vi "Correggi database tempo acq da hms.vi"() -> ()   [LabVIEW 2019]
uses:
  <vilib>/addons/database/Connection.llb/Conn Execute.vi
  <vilib>/addons/database/Recordset.llb/Rec Fetch Recordset Data (R).vi
  <vilib>/addons/database/Recordset.llb/Rec Destroy - Connection.vi
  <vilib>/addons/database/_DB Variant To Data/Database Variant To Data.xnode
  <vilib>/addons/database/NI_Database_API.lvlib
panel:
  in  "Tempo T\\corrente F":bool
  out "data 2":string[][](array[string])
  out "Numeric 2":i32
  out "concatenated string 2":string
  out "error out 2":errorcluster
  out "error out":errorcluster
  out "concatenated string":string
  out "Numeric":i32
  out "data":string[][](array[string])
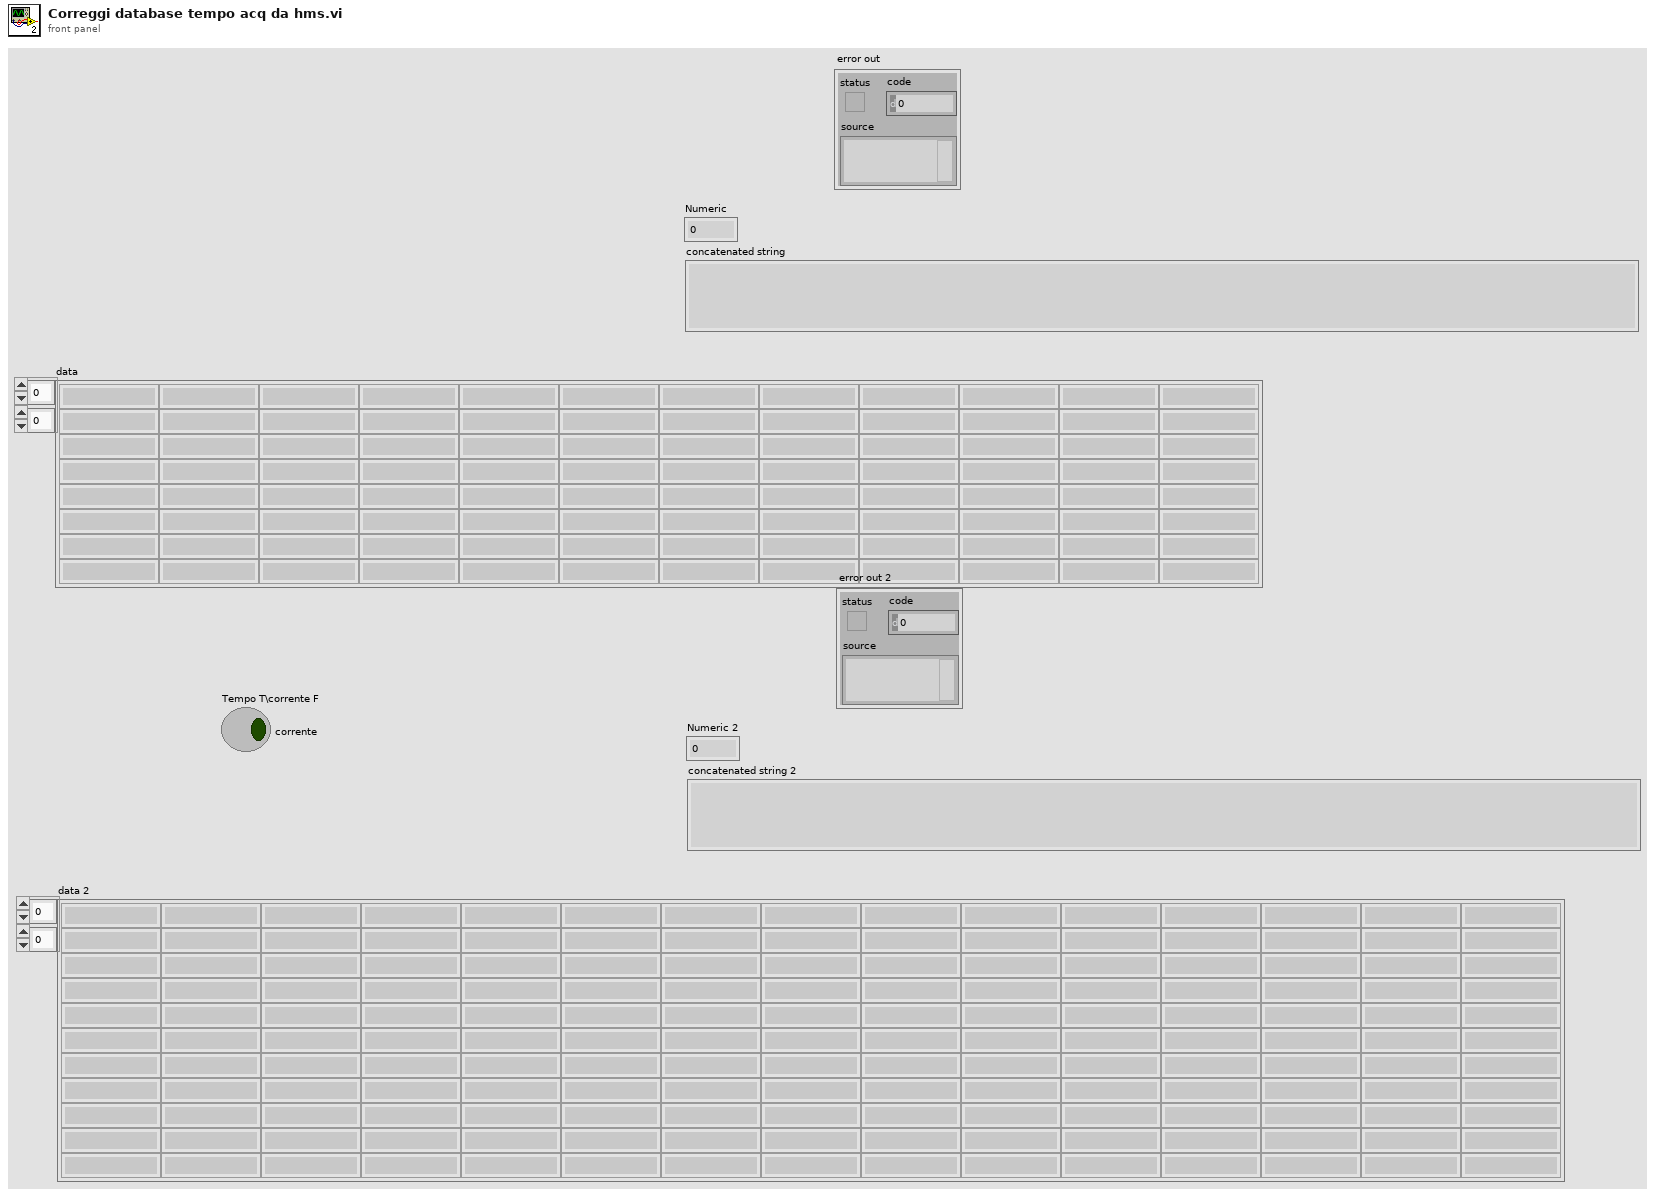
[diagram p1: front panel]
types:
  T1 = typedef "NI_Database_API.lvlib/Conn ObjectReference.ctl" = refnum<k1>
  T2 = typedef "NI_Database_API.lvlib/Rec ObjectReference.ctl" = refnum<k1>
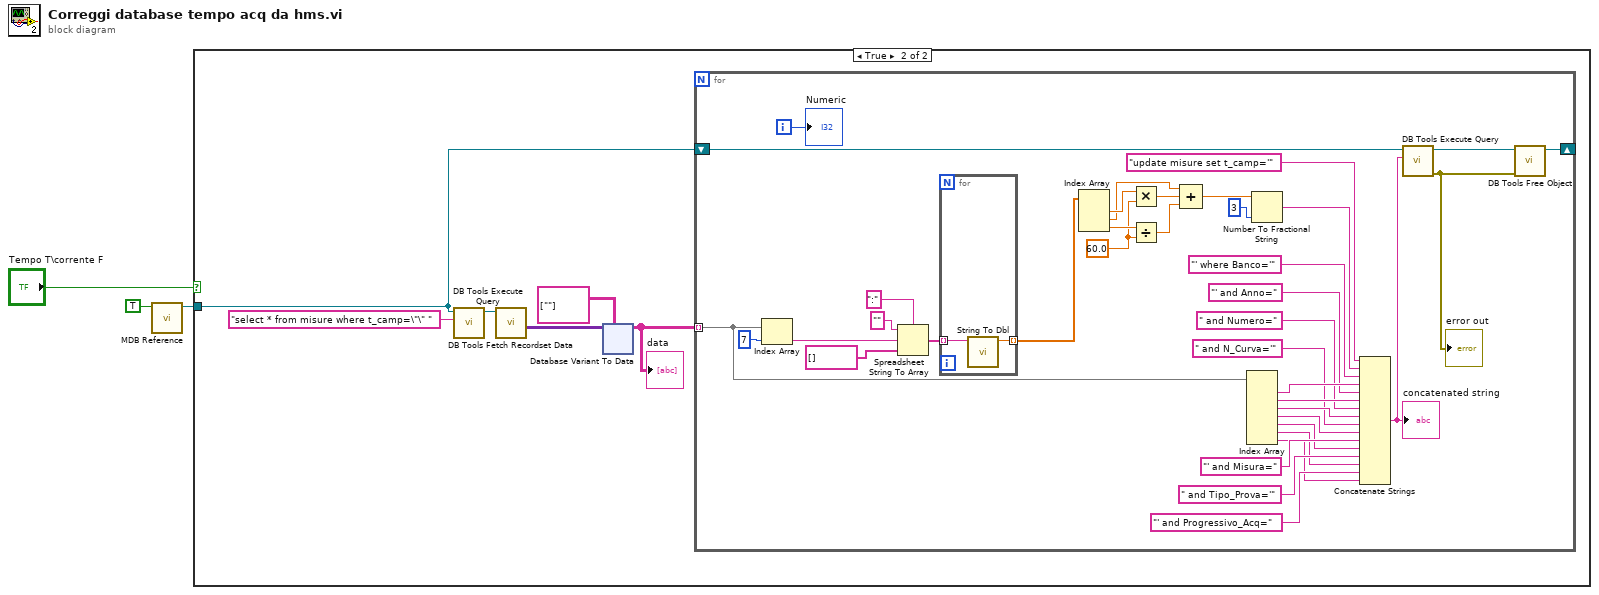
[diagram p0: block diagram]
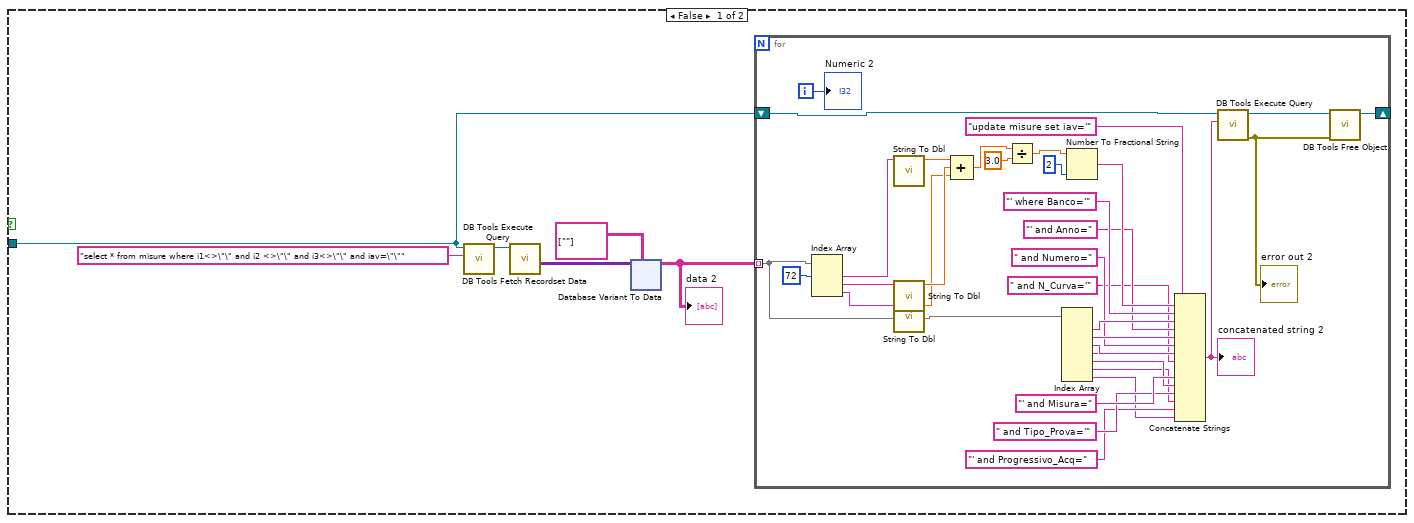
[diagram p2: hidden frame]
diagram:
  n1 = call "MDB Reference.vi"("Collaudi T/motori F"=TRUE) -> ("Refnum out"=w2:T1)  [unwired: 8 in, 2 out]
  n2 = case shown="True" "Tempo T\\corrente F" {
    tunnel: w2 -> [w4 w88]
    frame False {
      n3 = call-poly <vilib>:"DB Tools Execute Query.vi"("SQL query"="select * from misure where i1<>\"\" and i2 <>\"\" and i3<>\"\" and iav=\"\"", "connection reference"=w4) -> ("recordset reference"=w5:T2)  [unwired: 6 in, 1 out]
      n4 = call-poly <vilib>:"DB Tools Fetch Recordset Data.vi"("recordset reference"=w5) -> ("recordset data"=w9:variant[][])  [unwired: 4 in, 2 out]
      n5 = xnode "Database Variant To Data"("database variant"=w9, "type"=string[][] [[""]]) -> ("data"=w6:string[][])  [unwired: 1 in, 1 out]
      "data 2" <- w6
      n6 = for {
        tunnel: w6 -> [w41] mode=indexing
        shift-right: [w20] -> _
        shift-left: w4 -> [w24]
        i -> [w22]
        n7 = Index Array(array=w41, index #1=72 ("index")) -> (element #1=w18:string, element #2=w17:string, element #3=w16:string)  [unwired: 2 in]
        n8 = call "String To Dbl.vi"("String"=w18) -> ("Numeric"=w15:dbl)  [unwired: 10 in]
        n9 = call "String To Dbl.vi"("String"=w17) -> ("Numeric"=w14:dbl)  [unwired: 10 in]
        n10 = call "String To Dbl.vi"("String"=w16) -> ("Numeric"=w13:dbl)  [unwired: 10 in]
        n11 = Compound Arithmetic op=ADD(w15, w14, w13) -> (w12:dbl)
        n12 = Divide(x=w12, y=3.0) -> (x/y=w10:dbl)
        n13 = Index Array(array=w41) -> (element #1=w37:string, element #2=w35:string, element #3=w33:string, element #4=w31:string, element #5=w29:string, element #6=w27:string, element #7=w25:string)  [unwired: 7 in]
        n14 = Number To Fractional String(number=w10, precision (6)=i16 2) -> (F-format string=w39:string)  [unwired: 2 in]
        n15 = Concatenate Strings("update misure set iav='", w39, "' where Banco='" ("string"), w37, "' and Anno=" ("string"), w35, " and Numero=" ("string"), w33, " and N_Curva='" ("string"), w31, "' and Misura=" ("string"), w29, " and Tipo_Prova='" ("string"), w27, "' and Progressivo_Acq=" ("string"), w25) -> (w23:string)
        "concatenated string 2" <- w23
        n16 = call-poly <vilib>:"DB Tools Execute Query.vi"("SQL query"=w23, "connection reference"=w24) -> ("error out"=w19:errorcluster, "recordset reference"=w21:T2)  [unwired: 6 in]
        "error out 2" <- w19
        n17 = call-poly <vilib>:"DB Tools Free Object.vi"("error in (no error)"=w19, "recordset reference"=w21) -> ("connection reference"=w20:T1)  [unwired: 8 in, 1 out]
        "Numeric 2" <- w22
      }
    }
    frame True {
      n18 = call-poly <vilib>:"DB Tools Execute Query.vi"("SQL query"="select * from misure where t_camp=\"\" ", "connection reference"=w88) -> ("recordset reference"=w89:T2)  [unwired: 6 in, 1 out]
      n19 = call-poly <vilib>:"DB Tools Fetch Recordset Data.vi"("recordset reference"=w89) -> ("recordset data"=w93:variant[][])  [unwired: 4 in, 2 out]
      n20 = xnode "Database Variant To Data"("database variant"=w93, "type"=string[][] [[""]]) -> ("data"=w90:string[][])  [unwired: 1 in, 1 out]
      "data" <- w90
      n21 = for {
        tunnel: w90 -> [w116] mode=indexing
        shift-right: [w95] -> _
        shift-left: w88 -> [w99]
        i -> [w97]
        w120 = 60.0 ("y")
        n22 = Index Array(array=w116, index=7) -> (element=w129:string)
        n23 = Spreadsheet String To Array(delimiter (Tab)=":", format string="", spreadsheet string=w129, array type (2D Dbl)=string[] []) -> (array=w126:string[])
        n24 = for {
          tunnel: w126 -> [w133] mode=indexing
          tunnel: [w132] -> w125 mode=indexing
          n25 = call "String To Dbl.vi"("String"=w133) -> ("Numeric"=w132:dbl)  [unwired: 10 in]
        }
        n26 = Index Array(array=w125) -> (element #1=w124:dbl, element #2=w123:dbl, element #3=w121:dbl)  [unwired: 3 in]
        n27 = Multiply(x=w124, y=w120) -> (x*y=w122:dbl)
        n28 = Divide(x=w121, y=w120) -> (x/y=w119:dbl)
        n29 = Compound Arithmetic op=ADD(w123, w122, w119) -> (w118:dbl)
        n30 = Index Array(array=w116) -> (element #1=w112:string, element #2=w110:string, element #3=w108:string, element #4=w106:string, element #5=w104:string, element #6=w102:string, element #7=w100:string)  [unwired: 7 in]
        n31 = Number To Fractional String(number=w118, precision (6)=i16 3) -> (F-format string=w114:string)  [unwired: 2 in]
        n32 = Concatenate Strings("update misure set t_camp='", w114, "' where Banco='" ("string"), w112, "' and Anno=" ("string"), w110, " and Numero=" ("string"), w108, " and N_Curva='" ("string"), w106, "' and Misura=" ("string"), w104, " and Tipo_Prova='" ("string"), w102, "' and Progressivo_Acq=" ("string"), w100) -> (w98:string)
        "concatenated string" <- w98
        n33 = call-poly <vilib>:"DB Tools Execute Query.vi"("SQL query"=w98, "connection reference"=w99) -> ("error out"=w94:errorcluster, "recordset reference"=w96:T2)  [unwired: 6 in]
        "error out" <- w94
        n34 = call-poly <vilib>:"DB Tools Free Object.vi"("error in (no error)"=w94, "recordset reference"=w96) -> ("connection reference"=w95:T1)  [unwired: 8 in, 1 out]
        "Numeric" <- w97
      }
    }
  }
